vi "i2c_defs.vi"() -> ()   [LabVIEW 2013]
panel:
  in  "FPGA timer clock frequency":dbl=100000000.0 min=40000.0 max=2000000.0 format="%#_3p"
  in  "FPGA clock frequency":dbl=40000000.0 min=40000.0 max=2000000.0 format="%#_3p"
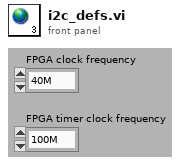
[diagram p1: front panel]
diagram:
